vi "SUB-Calculation_Scale_of_CDC.vi"(10 "MAX C":dbl format="%#.6g", 11 "MIN C":dbl format="%#.6g") -> (3 "Scale(CDC)":dbl format="%#.6g")   [LabVIEW 2015]
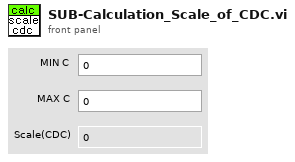
[diagram p1: front panel]
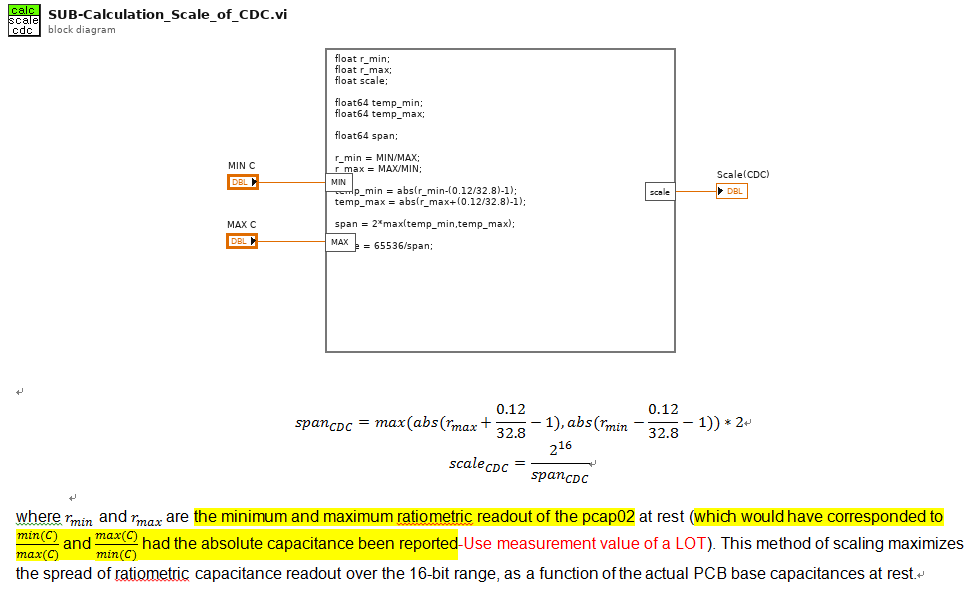
[diagram p0: block diagram]
diagram:
  n1 = formula code="float r_min;\nfloat r_max;\nfloat scale;\n\nfloat64 temp_min;\nfloat64 temp_max;\n\nfloat64 span;\n\nr_min = MIN/MAX;\nr_max = MAX/MIN;\n\ntemp_min = abs(r_min-(0.12/32.8)-1);\ntemp_max = abs(r_max+(0.12/32.8)-1);\n\nspan = 2*max(temp_min,temp_max);\n\nscale = 65536/span;"("MIN"="MIN C", "MAX"="MAX C") -> ("scale"=→"Scale(CDC)":dbl)
